vi "findProperties.vi"(8 "error in (no error)":errorcluster, 11 "IPropertyObject in":refnum<class "IPropertyObject.lvclass">) -> (0 "error out":errorcluster, 2 "Properties out":refnum<class "IProperty.lvclass">[](array[class]), 3 "IPropertyObject out":refnum<class "IPropertyObject.lvclass">)   [LabVIEW 2022 SP3, in "openDAQ.lvlib" / "IBaseObject.lvlib" / "IPropertyObject.lvlib" / "IPropertyObject.lvclass"]
uses:
  <instrlib>/openDAQ/Public/Classes/IPropertyObject/IPropertyObject.lvclass
  <instrlib>/openDAQ/Public/Classes/IPropertyObject/IPropertyObject.lvclass/IPropertyObject.ctl
  <instrlib>/openDAQ/Public/Classes/daqCoreTypes/IList/IList.lvclass
  <instrlib>/openDAQ/Public/Classes/daqCoreTypes/IList/Polymorphic/getList/getPropertyList.vi
  <instrlib>/openDAQ/Binaries/Windows/x86/copendaq32.dll
  <instrlib>/openDAQ/Public/Classes/IProperty/IProperty.lvclass
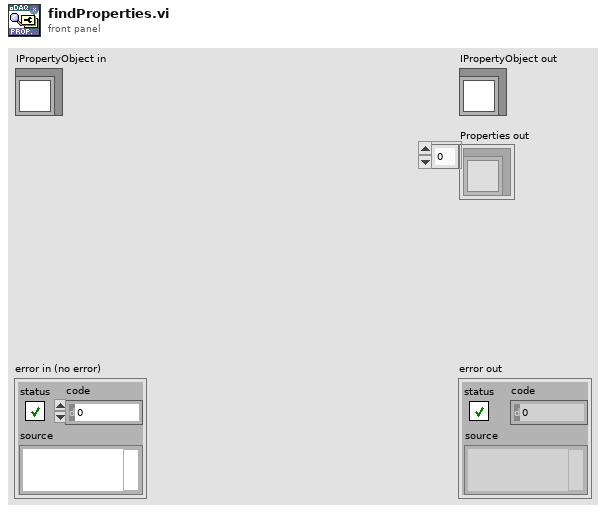
[diagram p1: front panel]
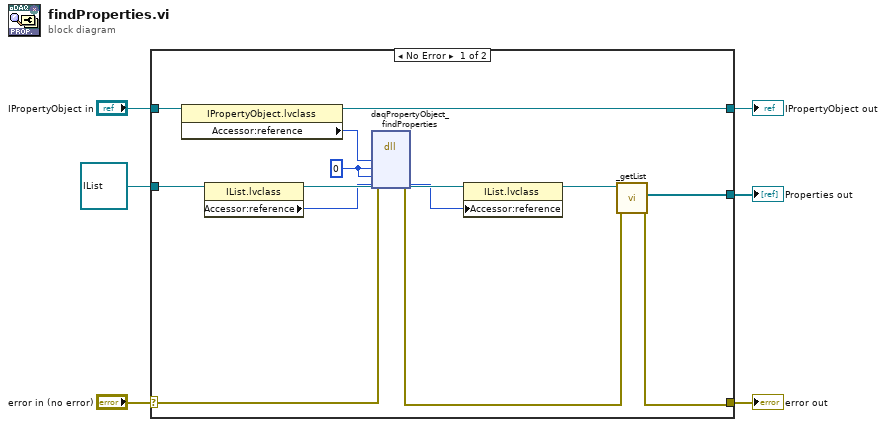
[diagram p0: block diagram]
diagram:
  n1 = case shown="No Error" "error in (no error)" {
    selector: "error in (no error)" -> [w12 w21]
    tunnel: [w8 w21] -> w5
    tunnel: [w17 w20] -> w3
    tunnel: "IPropertyObject in" -> [w18 w20]
    tunnel: refnum<class "IList.lvclass"> refnum ("openDAQ.lvlib:daqCoreTypes.lvlib:IList.lvclass") -> [w15 _]
    tunnel: [w10 _] -> w1
    frame No Error {
      w7 = i64 0 ("propertyFilter")
      n2 = property class="IPropertyObject.lvclass"(reference=w18) -> (reference out=w17:refnum<class "IPropertyObject.lvclass">, "Accessor:reference"=w16:i64)  [unwired: 1 in, 1 out]
      n3 = property class="IList.lvclass"(reference=w15) -> (reference out=w19:refnum<class "IList.lvclass">, "Accessor:reference"=w14:i64)  [unwired: 1 in, 1 out]
      n4 = dll-call lib="C:/Program Files (x86)/National Instruments/LabVIEW 2022/instr.lib/openDAQ/Binaries/Windows/x86/copendaq*.*" fn="daqPropertyObject_findProperties"(error in=w12, "propertyObject"=w16, "propertyFilter"=w7, "componentFilter"=w7, "visibleProperties"=w14) -> (error out=w9:errorcluster, "visibleProperties"=w13:i64)  [unwired: 6 in, 1 out]
      n5 = property class="IList.lvclass"(reference=w19, "Accessor:reference"=w13) -> (reference out=w11:refnum<class "IList.lvclass">)  [unwired: 1 in, 1 out]
      n6 = call-poly <instrlib>:"_getList.vi"("error in (no error)"=w9, "IList in"=w11) -> ("error out"=w8:errorcluster, "Properties out"=w10:refnum<class "IProperty.lvclass">[])  [unwired: 8 in]
    }
    frame Error {
    }
  }
  "error out" <- w5
  "IPropertyObject out" <- w3
  "Properties out" <- w1
